vi "S to T - 2nPort.vi"(8 "error in (no error)":errorcluster, 11 "S-par Array In":cdb[][](array[numeric])) -> (0 "error out":errorcluster, 3 "T-par Array Out":cdb[][](array[numeric]))   [LabVIEW 2023, in "NI_HFNetworkAnalysis.lvlib"]
doc: "Convert an S-parameters array of a 2n-port network to a T-parameters array:\n<b>{ b1, b2, ..., bn, a1, a2, an } = T . { an+1, an+2, ..., a2n, bn+1, bn+2, ..., b2n }</b>\n<b>{ b1, b2, ..., b2n } = S . { a1, a2, ..., a2n }</b>\n\nInput S-parameters array rows are defined as <b>(S11,S12,S13,S14,...,S21,S22,S23,S24,...,S31,S32,S33,S34,...,S41,S42,S43,S44,...)</b> \nand output T-parameters array rows are defined as <b>(T11,T12,T13,T14,...,T21,T22,T23,T24,...,T31,T32,T33,T34,...,T41,T42,T43,T44,...)</b>.\n\n<b>Note</b>\nThe convention for both S-parameters and T-parameters arrays for the current is <b>\"positive when flowing into the port\"</b>.\n\n<b>Known Limitations</b>\nTransformation supports only 2n-port networks."
uses:
  NI_HFNetworkAnalysis.lvlib
  <vilib>/Analysis/baseanly.llb/Complex A x B.vi
  <vilib>/Analysis/Matrix/Numeric/Conversions/Array To Matrix - CA2.vi
  <vilib>/Analysis/baseanly.llb/Complex Inverse Matrix.vi
  <vilib>/Analysis/Matrix/Numeric/Subtract/Subtract - CM,CM.vi
  <vilib>/Analysis/Matrix/Numeric/Conversions/Matrix To Array - CM.vi
  <vilib>/Analysis/Matrix/NI_Matrix.lvlib
  <vilib>/Analysis/NI_AALBase.lvlib
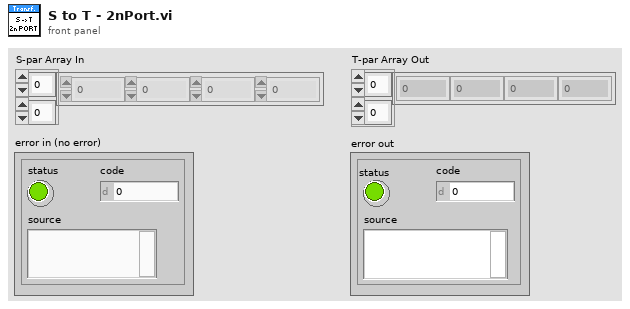
[diagram p1: front panel]
types:
  T1 = typedef "NI_Matrix.lvlib/ComplexMatrix.ctl" = cdb[][]
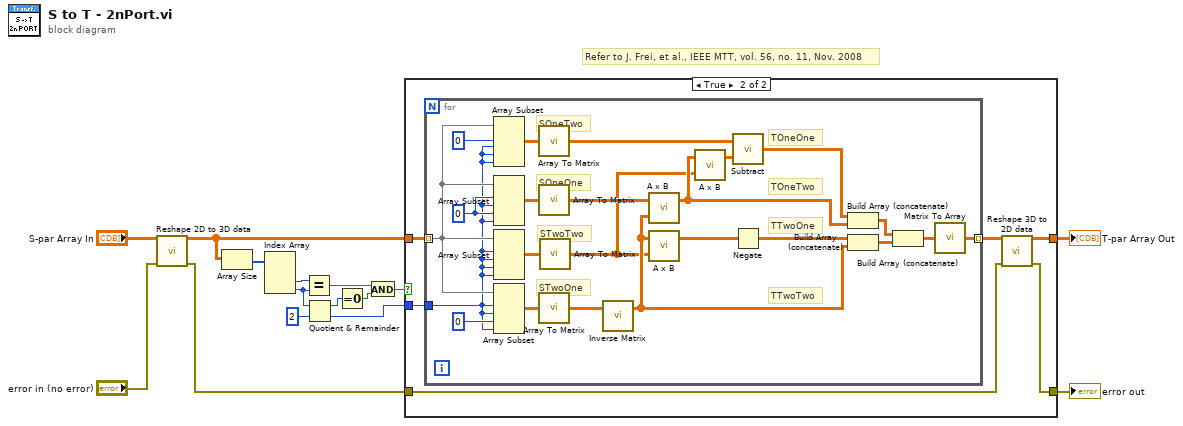
[diagram p0: block diagram]
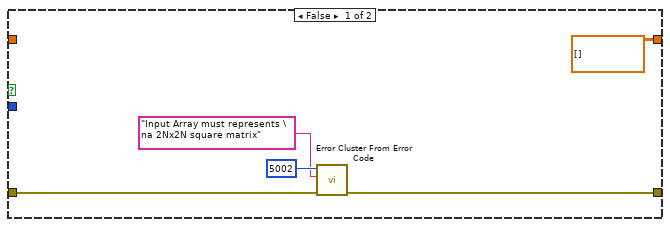
[diagram p2: hidden frame]
diagram:
  # "Refer to J. Frei, et al., IEEE MTT, vol. 56, no. 11, Nov. 2008"
  n1 = call "Reshape 2D to 3D data.vi"("Parameters In (2D)"="S-par Array In", "Error In"="error in (no error)") -> ("Parameters Out (3D)"=w14:cdb[][][], "Error Out"=w5:errorcluster)  [unwired: 12 in]
  n2 = Array Size(array=w14) -> (size(s)=w13:i32[])
  n3 = Index Array(array=w13) -> (element #2=w8:i32, element #3=w12:i32)  [unwired: 3 in, 1 out]
  n4 = Equal?(x=w8, y=w12) -> (x = y?=w10:bool)
  n5 = Quotient & Remainder(x=w12, y=2) -> (x-y*floor(x/y)=w2:i32, floor(x/y)=w1:i32)
  n6 = Equal To 0?(x=w2) -> (x = 0?=w9:bool)
  n7 = And(x=w10, y=w9) -> (x .and. y?=w7:bool)
  n8 = case shown="True" w7 {
    tunnel: w14 -> [_ w26]
    tunnel: w1 -> [_ w25]
    tunnel: [cdb[][] [] ("Parameters Out (2D)") w23] -> w6
    tunnel: w5 -> [w19 w22]
    tunnel: [w18 w21] -> w3
    frame False {
      n9 = call <vilib>:"Error Cluster From Error Code.vi"("error in (no error)"=w19, "error message (\"\")"="Input Array must represents \na 2Nx2N square matrix" ("error message (\"\")"), "error code (0)"=5002) -> ("error out"=w18:errorcluster)  [unwired: 6 in]
    }
    frame True {
      n10 = for {
        tunnel: w26 -> [w46] mode=indexing
        tunnel: w25 -> [w45]
        tunnel: [w27] -> w24 mode=indexing
        w49 = 0 ("index")
        # "TTwoOne"
        # "TOneTwo"
        # "TOneOne"
        # "TTwoTwo"
        # "STwoTwo"
        # "STwoOne"
        # "SOneTwo"
        # "SOneOne"
        n11 = Array Subset(array=w46, index (row)=0 ("index"), length (row)=w45, index (col)=w45, length (col)=w45) -> (w43:cdb[][])
        n12 = Array Subset(array=w46, index (row)=w49, length (row)=w45, index (col)=w49, length (col)=w45) -> (w44:cdb[][])
        n13 = Array Subset(array=w46, index (row)=w45, length (row)=w45, index (col)=w45, length (col)=w45) -> (w41:cdb[][])
        n14 = Array Subset(array=w46, index (row)=w45, length (row)=w45, index (col)=0 ("index"), length (col)=w45) -> (w42:cdb[][])
        n15 = call-poly <vilib>:"Array To Matrix.vi"("Complex 2D Array"=w43) -> ("Complex Matrix"=w38:T1)
        n16 = call-poly <vilib>:"Array To Matrix.vi"("Complex 2D Array"=w44) -> ("Complex Matrix"=w39:T1)
        n17 = call-poly <vilib>:"Array To Matrix.vi"("Complex 2D Array"=w42) -> ("Complex Matrix"=w40:T1)
        n18 = call-poly <vilib>:"Array To Matrix.vi"("Complex 2D Array"=w41) -> ("Complex Matrix"=w29:T1)
        n19 = call-poly <vilib>:"Inverse Matrix.vi"("Input Matrix"=w40) -> ("Inverse Matrix"=w30:T1)  [unwired: 1 in, 1 out]
        n20 = call-poly <vilib>:"A x B.vi"("B"=w30, "A"=w39) -> ("A x B"=w33:T1)  [unwired: 1 out]
        n21 = call-poly <vilib>:"A x B.vi"("B"=w29, "A"=w30) -> ("A x B"=w32:T1)  [unwired: 1 out]
        n22 = call-poly <vilib>:"A x B.vi"("B"=w29, "A"=w33) -> ("A x B"=w37:T1)  [unwired: 1 out]
        n23 = call-poly <vilib>:"Subtract.vi"("Complex Matrix B"=w37, "Complex Matrix A"=w38) -> ("A - B"=w34:T1)
        n24 = Negate(x=w32) -> (-x=w31:T1)
        n25 = Build Array (concatenate)(w34, w33) -> (w36:T1)
        n26 = Build Array (concatenate)(w31, w30) -> (w35:T1)
        n27 = Build Array (concatenate)(w36, w35) -> (w28:T1)
        n28 = call-poly <vilib>:"Matrix To Array.vi"("Complex Matrix"=w28) -> ("Complex 2D Array"=w27:cdb[][])
      }
      n29 = call "Reshape 3D to 2D data.vi"("Parameters In (3D)"=w24, "Error In"=w22) -> ("Parameters Out (2D)"=w23:cdb[][], "Error Out"=w21:errorcluster)  [unwired: 12 in]
    }
  }
  "T-par Array Out" <- w6
  "error out" <- w3
